vi "SwapInstanceVIUnusedName2 42.vi"(6 "Bindata & descr in":T1, 7 "type":i64, 8 "error in (no error)":errorcluster, 9 "dims":u8=3 min=1 max=3, 11 "kwarg_name":string="testarg") -> (0 "error out":errorcluster, 1 "Array 3D":i64[][][](array[numeric]), 2 "Array 2D":i64[][](array[numeric]), 3 "Array 1D":i64[](array[numeric]), 4 "Bindata & descr out":T1, 5 "bindata":u8[](array[numeric]))   [LabVIEW 2018]
uses:
  Bindata&description.ctl
  Bindata description.ctl
  236d3e0c-60a7-4ae5-9bc9-0ff41b983f05.vi
  b449f9df-ee8d-489b-9487-897c21ba14eb.vi
  e7b7674e-094d-4356-9454-cca6775f0358.vi
  025d52f7-3b03-4309-bff2-4ec84fc3d60c.vi
  b449f9df-ee8d-489b-9487-897c21ba14eb.vi/9a929507-b059-4abd-9ed4-ef53a005ff63.vi
  e7b7674e-094d-4356-9454-cca6775f0358.vi/ad73f5ce-7658-473b-b9fc-fac91a92da1e.vi
  025d52f7-3b03-4309-bff2-4ec84fc3d60c.vi/5d27c3aa-c82a-4d9f-96ad-8781e4a71ba1.vi
  b449f9df-ee8d-489b-9487-897c21ba14eb.vi/9a929507-b059-4abd-9ed4-ef53a005ff63.vi/47391a1c-e85f-44cf-90f5-ee97f4b4554e.vi
  e7b7674e-094d-4356-9454-cca6775f0358.vi/ad73f5ce-7658-473b-b9fc-fac91a92da1e.vi/6213ee20-5898-4e73-9fb0-a99b3c67ea96.vi
  025d52f7-3b03-4309-bff2-4ec84fc3d60c.vi/5d27c3aa-c82a-4d9f-96ad-8781e4a71ba1.vi/cb9fe9ca-b60f-4580-8939-faeac5c9a8ca.vi
  b449f9df-ee8d-489b-9487-897c21ba14eb.vi/9a929507-b059-4abd-9ed4-ef53a005ff63.vi/47391a1c-e85f-44cf-90f5-ee97f4b4554e.vi/32eb32a5-6c8c-4395-ad45-adfd19c3e226.vi
  e7b7674e-094d-4356-9454-cca6775f0358.vi/ad73f5ce-7658-473b-b9fc-fac91a92da1e.vi/6213ee20-5898-4e73-9fb0-a99b3c67ea96.vi/ff21df5d-9d2e-4549-80bf-e7815593682d.vi
  025d52f7-3b03-4309-bff2-4ec84fc3d60c.vi/5d27c3aa-c82a-4d9f-96ad-8781e4a71ba1.vi/cb9fe9ca-b60f-4580-8939-faeac5c9a8ca.vi/41816769-e1ec-46ec-9aae-7d6f9525b3ed.vi
  check ID validity.vi
  LV-Julia_ZMQ-Roundtrip_lib.lvlib
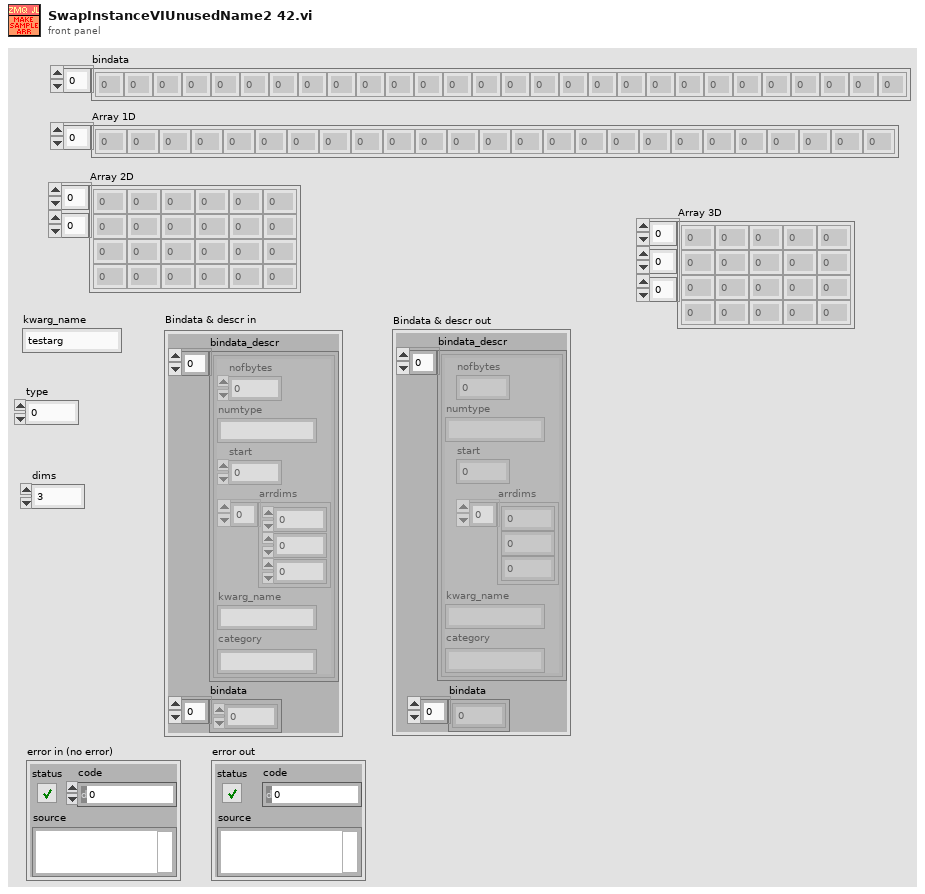
[diagram p1: front panel]
types:
  T1 = typedef "Bindata&description.ctl" = cluster{"bindata_descr":T2[], "bindata":u8[]}
  T2 = typedef "LV-Julia_ZMQ-Roundtrip_lib.lvlib/Bindata description.ctl" = cluster{"nofbytes":i32, "numtype":string, "start":i32, "arrdims":i32[], "kwarg_name":string, "category":string}
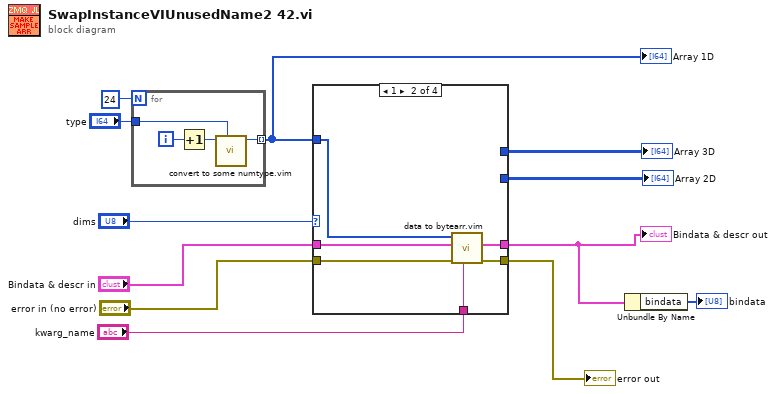
[diagram p0: block diagram]
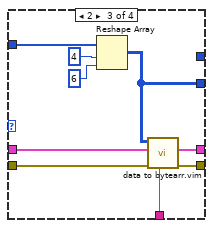
[diagram p3: hidden frame]
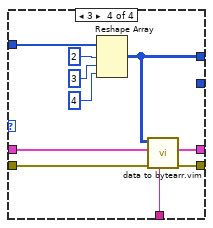
[diagram p4: hidden frame]
diagram:
  n1 = for {
    N: 24 -> [_]
    tunnel: [w14] -> w11 mode=indexing
    tunnel: "type" -> [w13]
    i -> [w16]
    n2 = Increment(x=w16) -> (x+1=w15:i32)
    n3 = call "convert to some numtype.vim"("type"=w13, "Numeric in"=w15) -> ("Numeric out"=w14:i64)  [unwired: 9 in]
  }
  "Array 1D" <- w11
  n4 = case shown="1" "dims" {
    tunnel: [_ _ _ w42] -> w12
    tunnel: w11 -> [_ w23 w30 w38]
    tunnel: "kwarg_name" -> [_ w22 w29 w37]
    tunnel: "error in (no error)" -> [w17 w21 w28 w36]
    tunnel: [w17 w20 w27 w35] -> w5
    tunnel: [_ w19 w26 w34] -> w2
    tunnel: [_ _ w25 _] -> w4
    tunnel: "Bindata & descr in" -> [_ w18 w24 w33]
    frame 0, Default {
    }
    frame 1 {
      n5 = call "data to bytearr.vim"("kwarg_name"=w22, "error in (no error)"=w21, "Bindata & descr in"=w18, "data in"=w23) -> ("error out"=w20:errorcluster, "Bindata & descr out"=w19:T1)  [unwired: 5 in, 1 out]
    }
    frame 2 {
      n6 = Reshape Array(w30, 4 ("dimension size"), 6 ("dimension size")) -> (w25:i64[][])
      n7 = call "data to bytearr.vim"("kwarg_name"=w29, "error in (no error)"=w28, "Bindata & descr in"=w24, "data in"=w25) -> ("error out"=w27:errorcluster, "Bindata & descr out"=w26:T1)  [unwired: 5 in, 1 out]
    }
    frame 3 {
      n8 = Reshape Array(w38, 2 ("dimension size"), 3 ("dimension size"), 4 ("dimension size")) -> (w42:i64[][][])
      n9 = call "data to bytearr.vim"("kwarg_name"=w37, "error in (no error)"=w36, "Bindata & descr in"=w33, "data in"=w42) -> ("error out"=w35:errorcluster, "Bindata & descr out"=w34:T1)  [unwired: 5 in, 1 out]
    }
  }
  "Array 3D" <- w12
  "Bindata & descr out" <- w2
  "error out" <- w5
  "Array 2D" <- w4
  n10 = Unbundle By Name(w2) -> ("bindata"=→"bindata":u8[])
